vi "Set ICAN.vi"(10 "ICAN":refnum<class "ICAN.lvclass">, 11 "CAN Task in":refnum<class "CAN Task.lvclass">) -> (3 "CAN Task out":refnum<class "CAN Task.lvclass">)   [LabVIEW 2024, in "canopen.lvlib" / "CAN Task.lvlib" / "CAN Task.lvclass"]
uses:
  CAN Task.lvclass
  CAN Task.lvclass/CAN Task.ctl
  HAL/HAL/Protocols/ICAN/ICAN.lvclass
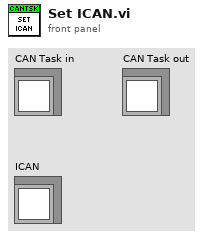
[diagram p1: front panel]
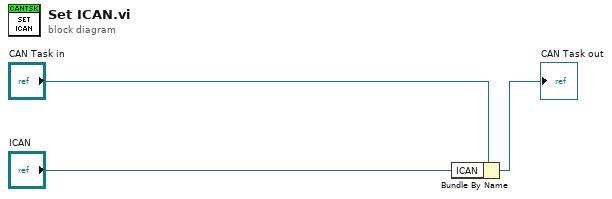
[diagram p0: block diagram]
diagram:
  n1 = Bundle By Name(cluster="CAN Task in", "ICAN"="ICAN") -> (→"CAN Task out":refnum<class "CAN Task.lvclass">)
